vi "Incubator Stretching - Both Channel Outputs.vi"() -> ()   [LabVIEW 2020]
panel:
  in  "stop":bool
  out "error out 2":errorcluster
  in  "Channel (1/2) 2":i32=1
  in  "OFF      ON":bool
  in  "Off time (s) 2":dbl
  in  "On time (s) 2":dbl
  in  "Current (A) 2":dbl
  in  "Voltage (V) 2":dbl
  in  "Channel (1/2)":i32=1
  in  "OFF      ON":bool
  in  "Off time (s)":dbl
  in  "On time (s)":dbl
  in  "Current (A)":dbl
  in  "Voltage (V)":dbl
  out "error out":errorcluster
  in  "error in (no error)":errorcluster
  in  "VISA resource name - Instrument Identifier":refnum<visa-resource-name>
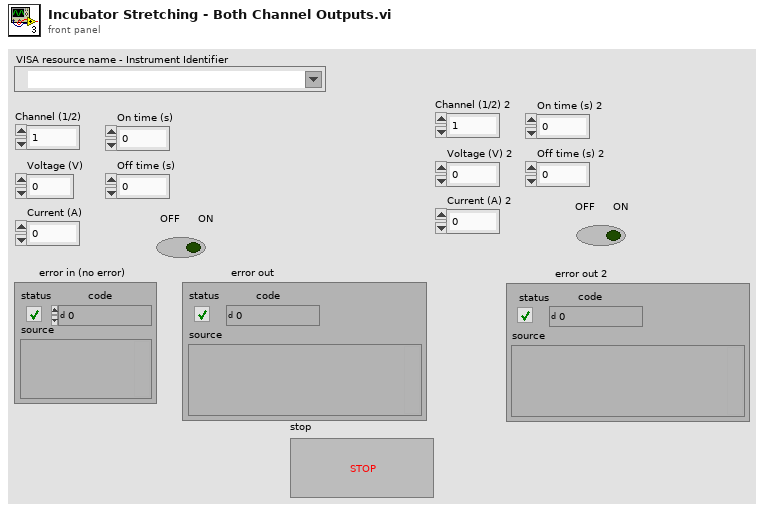
[diagram p1: front panel]
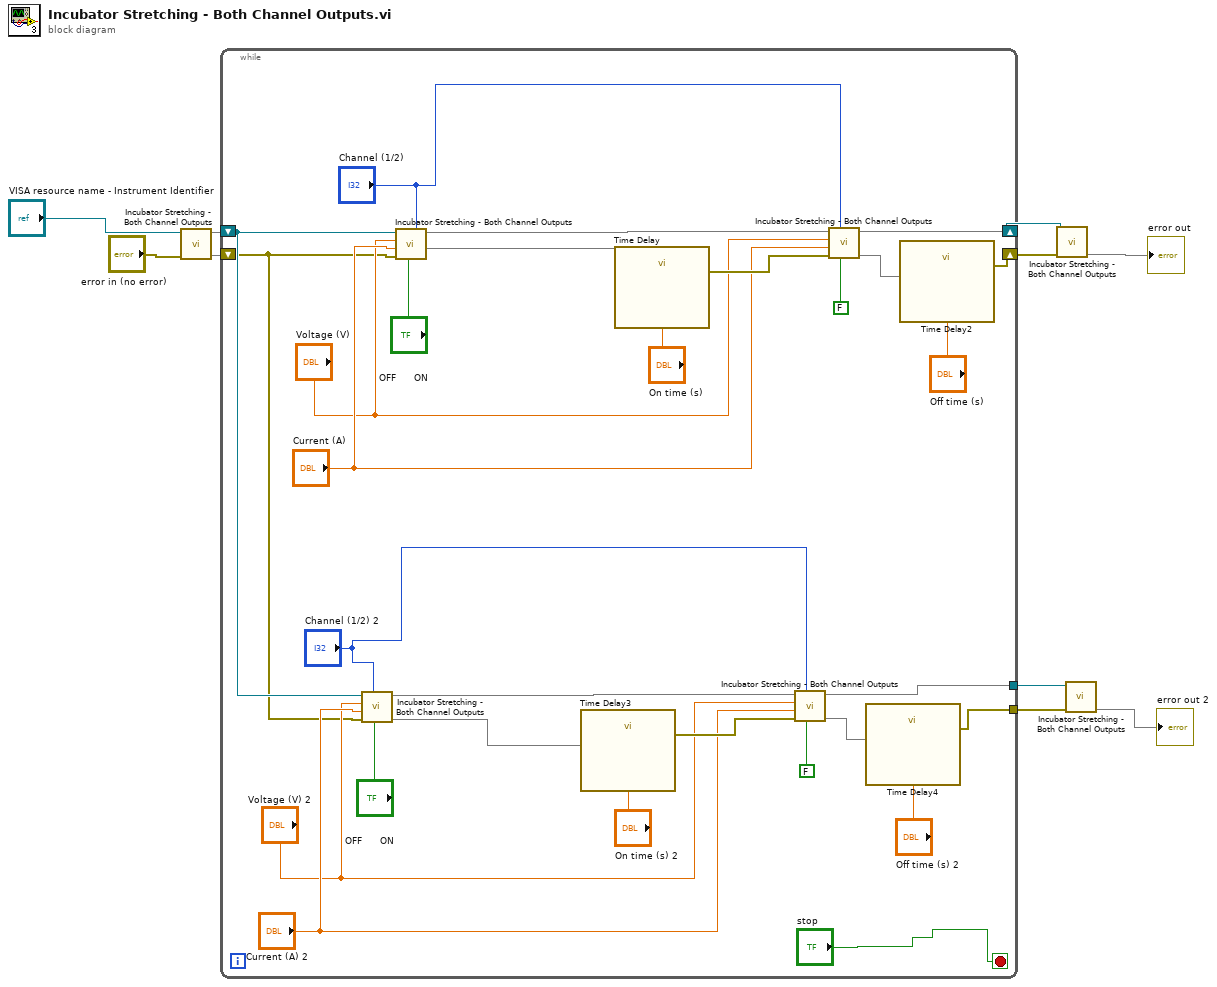
[diagram p0: block diagram]
diagram:
  n1 = call "Incubator Stretching - Both Channel Outputs.vi"(8:"error in (no error)", 11:"VISA resource name - Instrument Identifier") -> (0:w6, 3:w7)  [unwired: 8 in]
  n2 = while {
    tunnel: [w17] -> w3
    tunnel: [w16] -> w1
    shift-right: [w18] -> w5
    shift-left: w7 -> [w21]
    shift-right: [w34] -> w8
    shift-left: w6 -> [w19]
    stop <- "stop" stop-if-true
    n3 = call "Incubator Stretching - Both Channel Outputs.vi"(6:"OFF      ON", 7:"Channel (1/2) 2", 8:w19, 9:"Current (A) 2", 10:"Voltage (V) 2", 11:w21) -> (0:w11, 3:w12)  [unwired: 4 in]
    n4 = call "Incubator Stretching - Both Channel Outputs.vi"(6:"OFF      ON", 7:"Channel (1/2)", 8:w19, 9:"Current (A)", 10:"Voltage (V)", 11:w21) -> (0:w13, 3:w14)  [unwired: 4 in]
    n5 = call "Time Delay3"("error in (no error)"=w11, "Delay Time (s)"="On time (s) 2") -> ("error out"=w28:errorcluster)  [unwired: 9 in]
    n6 = call "Time Delay"("error in (no error)"=w13, "Delay Time (s)"="On time (s)") -> ("error out"=w38:errorcluster)  [unwired: 9 in]
    n7 = call "Incubator Stretching - Both Channel Outputs.vi"(6:FALSE, 7:"Channel (1/2) 2", 8:w28, 9:"Current (A) 2", 10:"Voltage (V) 2", 11:w12) -> (0:w26, 3:w16)  [unwired: 4 in]
    n8 = call "Incubator Stretching - Both Channel Outputs.vi"(6:FALSE, 7:"Channel (1/2)", 8:w38, 9:"Current (A)", 10:"Voltage (V)", 11:w14) -> (0:w35, 3:w18)  [unwired: 4 in]
    n9 = call "Time Delay4"("error in (no error)"=w26, "Delay Time (s)"="Off time (s) 2") -> ("error out"=w17:errorcluster)  [unwired: 9 in]
    n10 = call "Time Delay2"("error in (no error)"=w35, "Delay Time (s)"="Off time (s)") -> ("error out"=w34:errorcluster)  [unwired: 9 in]
  }
  n11 = call "Incubator Stretching - Both Channel Outputs.vi"(8:w8, 11:w5) -> (0:→"error out")  [unwired: 9 in]
  n12 = call "Incubator Stretching - Both Channel Outputs.vi"(8:w3, 11:w1) -> (0:→"error out 2")  [unwired: 9 in]
